vi "UL SAVE MEI.vi"(6 "Slide in":refnum<vi>, 7 "NM?":bool, 8 "error out IN":errorcluster, 9 "ItemNames":string[][](array[string]), 10 "Array vf":bool[][][](array[boolean]), 11 "Array MEMO":string[][][](array[string])) -> (0 "error out":errorcluster)   [LabVIEW 2019]
uses:
  <vilib>/addons/database/NI_Database_API.lvlib
panel:
  out "x+y 2":dbl
  out "x+y":dbl
  in  "stop":bool
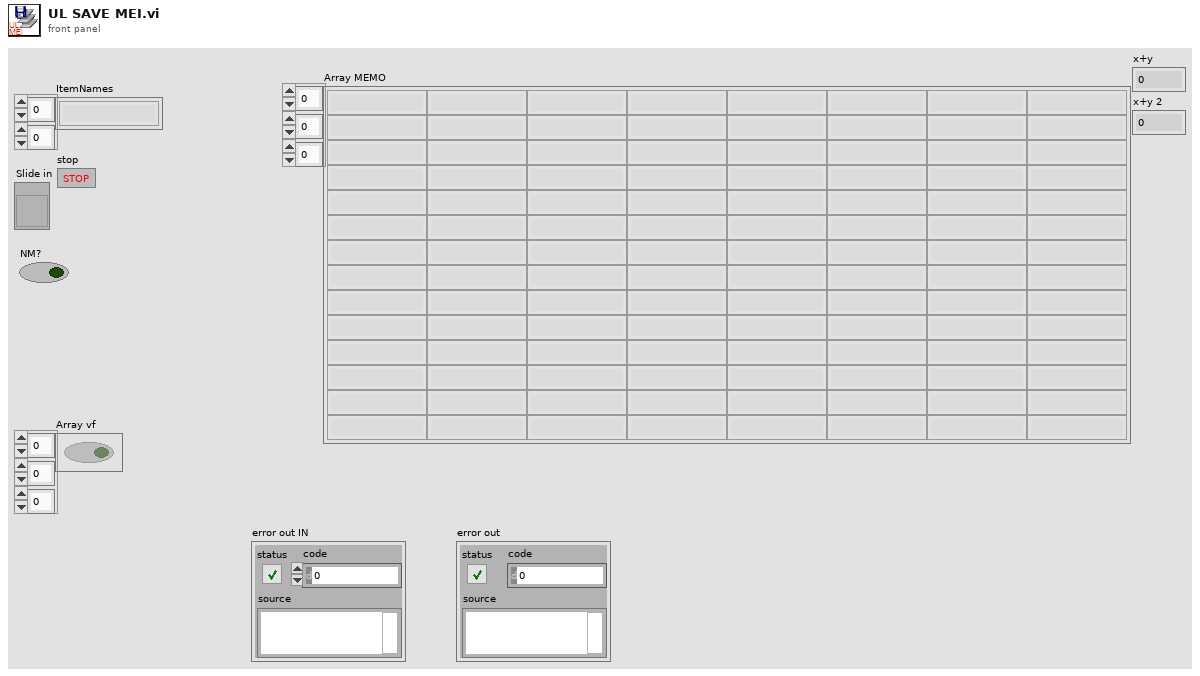
[diagram p1: front panel]
types:
  T1 = cluster{"Array of elements":cluster{"String":string, "variant":variant}[], "Single element":cluster{"String":string, "variant":variant}, "enque at\nopposite end (F)":bool, "no replications (F)":bool}
  T2 = typedef "NI_Database_API.lvlib/Conn ObjectReference.ctl" = refnum<k1>
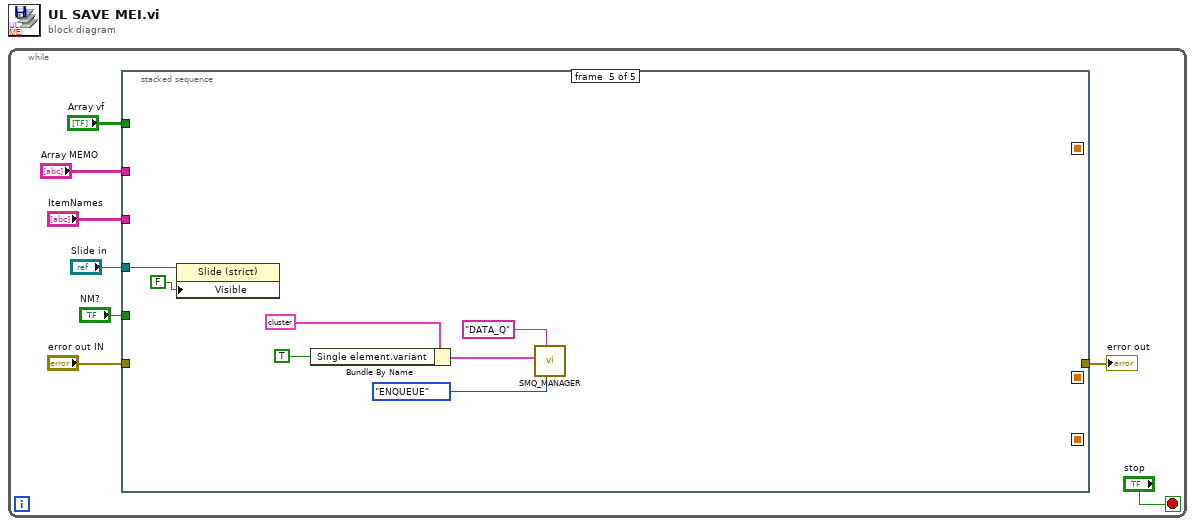
[diagram p0: block diagram]
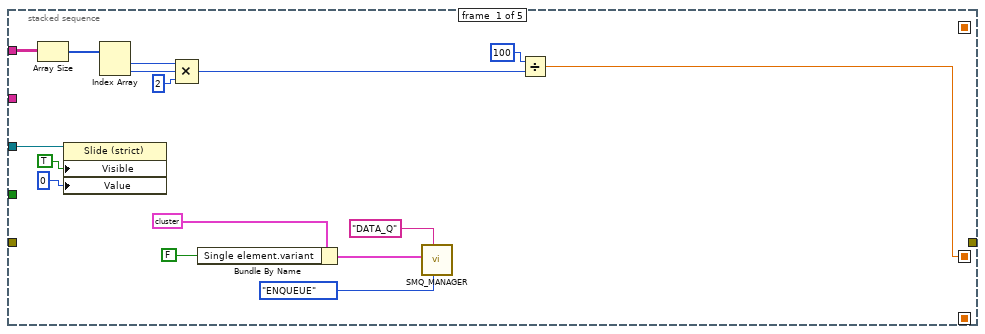
[diagram p2: hidden frame]
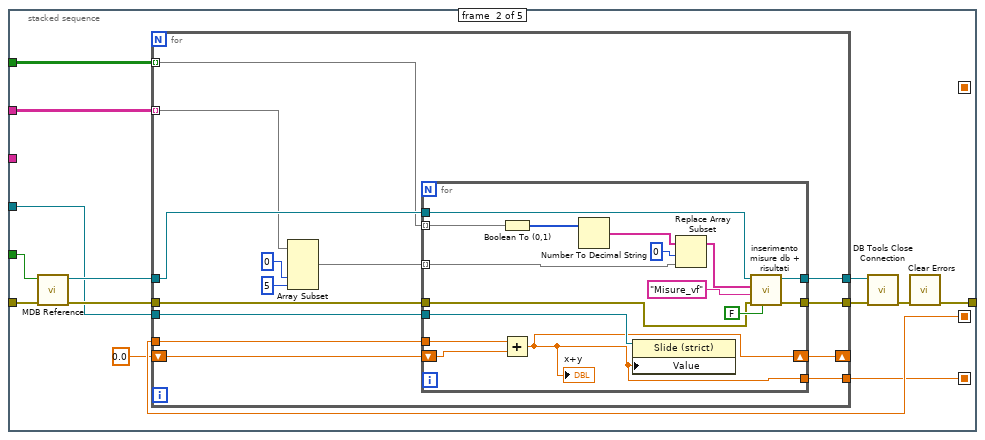
[diagram p3: hidden frame]
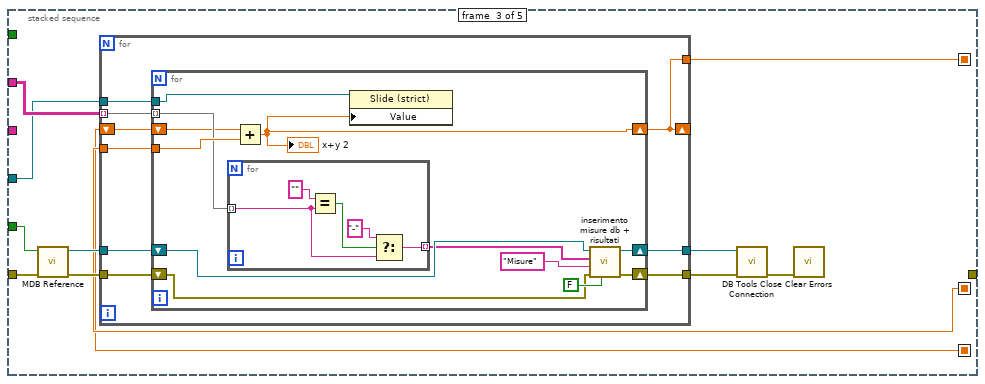
[diagram p4: hidden frame]
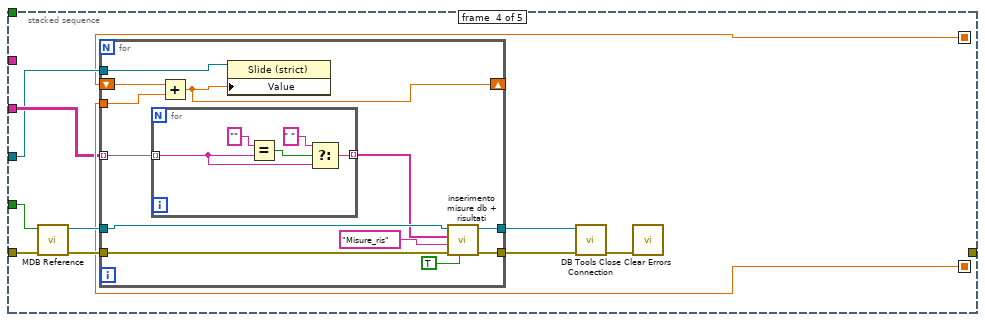
[diagram p5: hidden frame]
diagram:
  n1 = while {
    stop <- "stop" stop-if-true
    n2 = stacked-sequence {
      seq-local: [w12 _ _ _ _] -> [_ w31 w74 w112 _]
      seq-local: [_ w26 _ _ _] -> [_ _ w70 _ _]
      seq-local: [_ _ w69 _ _] -> [_ _ _ w107 _]
      tunnel: "Array MEMO" -> [w19 w32 w75 _ _]
      tunnel: "Array vf" -> [_ w34 _ _ _]
      tunnel: "NM?" -> [_ w38 w80 w117 _]
      tunnel: [_ w27 _ _ _] -> w7
      tunnel: "ItemNames" -> [_ _ _ w111 _]
      tunnel: "Slide in" -> [w10 w30 w73 w110 w135]
      tunnel: "error out IN" -> [_ w29 w72 w109 _]
      frame #0 {
        n3 = Array Size(array=w19) -> (size(s)=w18:i32[])
        n4 = property on="Property Node" class="Slide (strict)"(reference=w10, "Visible"=TRUE, "Value"=u8 0) -> ()  [unwired: 1 in, 2 out]
        n5 = Index Array(array=w18) -> (element #1=w17:i32, element #2=w16:i32)  [unwired: 2 in]
        n6 = Compound Arithmetic op=MULTIPLY(w17, w16, 2 ("value")) -> (w13:i32)
        n7 = Bundle By Name(cluster=T1 {"Array of elements"=[], "Single element"={"String"="SEND MAIN2?", "variant"=variant}, "enque at\nopposite end (F)"=FALSE, "no replications (F)"=FALSE} ("Enqueue cluster"), "Single element.variant"=FALSE) -> (w20:T1)
        n8 = call <userlib>:"SMQ_MANAGER.vi"("Function"=enum16{"INITIALIZE", "ENQUEUE", "STOP ALL"}."ENQUEUE", "Queue name"="DATA_Q", "Enqueue cluster"=w20) -> ()  [unwired: 8 in, 1 out]
        n9 = Divide(x=100, y=w13) -> (x/y=w12:dbl)
      }
      frame #1 {
        n10 = call "MDB Reference.vi"("error in (no error)"=w29, "Collaudi T/motori F"=w38) -> ("error out"=w33:errorcluster, "Refnum out"=w37:T2)  [unwired: 7 in, 1 out]
        n11 = for {
          tunnel: w37 -> [w52]
          tunnel: [w51] -> w36
          tunnel: [w50] -> w35
          tunnel: w34 -> [w49] mode=indexing
          tunnel: w32 -> [w47] mode=indexing
          tunnel: w33 -> [w44]
          tunnel: w31 -> [w43]
          tunnel: w30 -> [w42]
          tunnel: [w41] -> w26
          shift-right: [w40] -> _
          shift-left: 0.0 -> [w39]
          n12 = Array Subset "Array Subset"(array=w47, index (col)=0 ("index"), length (col)=5 ("length")) -> (w45:string[][])  [unwired: 2 in]
          n13 = for {
            tunnel: [w64] -> w50
            tunnel: w52 -> [w68]
            tunnel: [w66] -> w51
            tunnel: w49 -> [w59] mode=indexing
            tunnel: w45 -> [w62] mode=indexing
            tunnel: w44 -> [w60]
            tunnel: w43 -> [w55]
            tunnel: w42 -> [w56]
            tunnel: [w54] -> w41
            shift-right: [w54] -> w40
            shift-left: w39 -> [w53]
            n14 = Boolean To (0,1)(Boolean=w59) -> (0, 1=w58:i16[])
            n15 = Add(x=w55, y=w53) -> (x+y=w54:dbl)
            "x+y" <- w54
            n16 = Number To Decimal String(number=w58) -> (decimal integer string=w57:string[])  [unwired: 1 out]
            n17 = property on="Property Node" class="Slide (strict)"(reference=w56, "Value"=w54) -> ()  [unwired: 1 in, 2 out]
            n18 = Replace Array Subset(array=w57, new element=w62, index=0) -> (w61:string[])
            n19 = call "inserimento misure db + risultati.vi"("Risultati?"=FALSE, "error out in"=w60, "nome tabella"="Misure_vf", "Risultati"=w61, "connection reference"=w68) -> ("error out"=w64:errorcluster, "connection reference out"=w66:T2)  [unwired: 4 in, 1 out]
          }
        }
        n20 = call <vilib>:"DB Tools Close Connection.vi"("error in (no error)"=w35, "connection reference"=w36) -> ("error out"=w28:errorcluster)  [unwired: 5 in]
        n21 = call <vilib>:"Clear Errors.vi"("error in (no error)"=w28) -> ("error out"=w27:errorcluster)  [unwired: 5 in, 1 out]
      }
      frame #2 {
        n22 = call "MDB Reference.vi"("error in (no error)"=w72, "Collaudi T/motori F"=w80) -> ("error out"=w76:errorcluster, "Refnum out"=w79:T2)  [unwired: 7 in, 1 out]
        n23 = for {
          tunnel: w79 -> [w89]
          tunnel: w75 -> [w88] mode=indexing
          tunnel: [w87] -> w78
          tunnel: [w86] -> w77
          tunnel: w76 -> [w85]
          tunnel: w74 -> [w84]
          tunnel: w73 -> [w83]
          shift-right: [w81] -> _
          shift-left: w70 -> [w82]
          tunnel: [w81] -> w69
          n24 = for {
            tunnel: w88 -> [w95] mode=indexing
            shift-right: [w99] -> w87
            shift-left: w89 -> [w101]
            shift-right: [w93] -> w86
            shift-left: w85 -> [w97]
            tunnel: w84 -> [w96]
            tunnel: w83 -> [w92]
            shift-right: [w90] -> w81
            shift-left: w82 -> [w91]
            n25 = for {
              tunnel: w95 -> [w104] mode=indexing
              tunnel: [w102] -> w94 mode=indexing
              n26 = Equal?(x="", y=w104) -> (x = y?=w105:bool)
              n27 = Select(t="-", s=w105, f=w104) -> (s? t:f=w102:string)
            }
            n28 = Add(x=w91, y=w96) -> (x+y=w90:dbl)
            "x+y 2" <- w90
            n29 = property on="Property Node" class="Slide (strict)"(reference=w92, "Value"=w90) -> ()  [unwired: 1 in, 2 out]
            n30 = call "inserimento misure db + risultati.vi"("Risultati?"=FALSE, "error out in"=w97, "nome tabella"="Misure", "Risultati"=w94, "connection reference"=w101) -> ("error out"=w93:errorcluster, "connection reference out"=w99:T2)  [unwired: 4 in, 1 out]
          }
        }
        n31 = call <vilib>:"DB Tools Close Connection.vi"("error in (no error)"=w77, "connection reference"=w78) -> ("error out"=w71:errorcluster)  [unwired: 5 in]
        n32 = call <vilib>:"Clear Errors.vi"("error in (no error)"=w71) -> ()  [unwired: 5 in, 2 out]
      }
      frame #3 {
        n33 = call "MDB Reference.vi"("error in (no error)"=w109, "Collaudi T/motori F"=w117) -> ("error out"=w113:errorcluster, "Refnum out"=w116:T2)  [unwired: 7 in, 1 out]
        n34 = for {
          tunnel: w116 -> [w129]
          tunnel: w111 -> [w122] mode=indexing
          tunnel: [w127] -> w115
          tunnel: [w125] -> w114
          tunnel: w113 -> [w124]
          tunnel: w112 -> [w123]
          tunnel: w110 -> [w120]
          shift-right: [w118] -> _
          shift-left: w107 -> [w119]
          n35 = for {
            tunnel: w122 -> [w132] mode=indexing
            tunnel: [w130] -> w121 mode=indexing
            n36 = Equal?(x="", y=w132) -> (x = y?=w133:bool)
            n37 = Select(t=" ", s=w133, f=w132) -> (s? t:f=w130:string)
          }
          n38 = Add(x=w119, y=w123) -> (x+y=w118:dbl)
          n39 = property on="Property Node" class="Slide (strict)"(reference=w120, "Value"=w118) -> ()  [unwired: 1 in, 2 out]
          n40 = call "inserimento misure db + risultati.vi"("Risultati?"=TRUE, "error out in"=w124, "nome tabella"="Misure_ris", "Risultati"=w121, "connection reference"=w129) -> ("error out"=w125:errorcluster, "connection reference out"=w127:T2)  [unwired: 4 in, 1 out]
        }
        n41 = call <vilib>:"DB Tools Close Connection.vi"("error in (no error)"=w114, "connection reference"=w115) -> ("error out"=w108:errorcluster)  [unwired: 5 in]
        n42 = call <vilib>:"Clear Errors.vi"("error in (no error)"=w108) -> ()  [unwired: 5 in, 2 out]
      }
      frame #4 {
        n43 = property on="Property Node" class="Slide (strict)"(reference=w135, "Visible"=FALSE) -> ()  [unwired: 1 in, 2 out]
        n44 = Bundle By Name(cluster=T1 {"Array of elements"=[], "Single element"={"String"="SEND MAIN2?", "variant"=variant}, "enque at\nopposite end (F)"=FALSE, "no replications (F)"=FALSE} ("Enqueue cluster"), "Single element.variant"=TRUE) -> (w137:T1)
        n45 = call <userlib>:"SMQ_MANAGER.vi"("Function"=enum16{"INITIALIZE", "ENQUEUE", "STOP ALL"}."ENQUEUE", "Queue name"="DATA_Q", "Enqueue cluster"=w137) -> ()  [unwired: 8 in, 1 out]
      }
    }
    "error out" <- w7
  }
